vi "GetFunctionConfig.vi"(8 "error in (no error)":errorcluster, 11 "FunctionBase In":refnum<class "FunctionBase.lvclass">) -> (0 "error out":errorcluster, 2 "FunctionConfig":variant, 3 "FunctionBase Out":refnum<class "FunctionBase.lvclass">)   [LabVIEW 2018, in "Functions.lvlib" / "FunctionBase.lvclass"]
uses:
  FunctionBase.lvclass
  <userlib>/NIST/BaseClasses/Object_class/BaseObject.lvclass
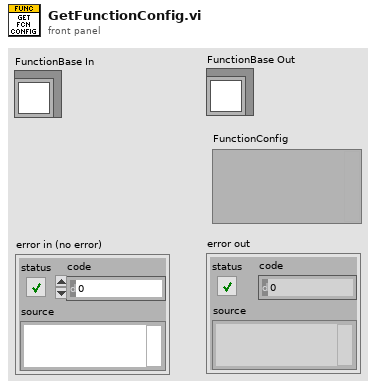
[diagram p1: front panel]
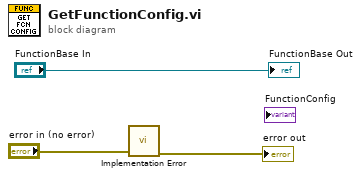
[diagram p0: block diagram]
diagram:
  n1 = call <userlib>:"Implementation Error.vi"("error in (no error)"="error in (no error)") -> ("error out"=→"error out":errorcluster)  [unwired: 10 in]
  "FunctionBase Out" <- "FunctionBase In"
